vi "DQMH_API_OpenCreateEventDialog.vi"(8 "error in (no error)":errorcluster) -> (0 "error out":errorcluster, 3 "DqmhCreateEventDialogRef":refnum<vi>, 5 "ApplicationRef":refnum<vi>)   [LabVIEW 2016]
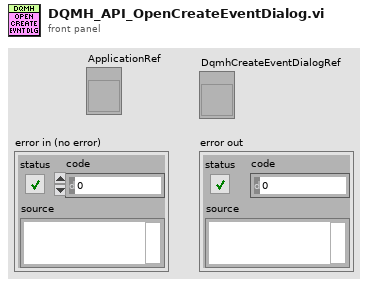
[diagram p1: front panel]
types:
  T1 = enum32{"Bad", "Idle", "Run top level", "Running"}
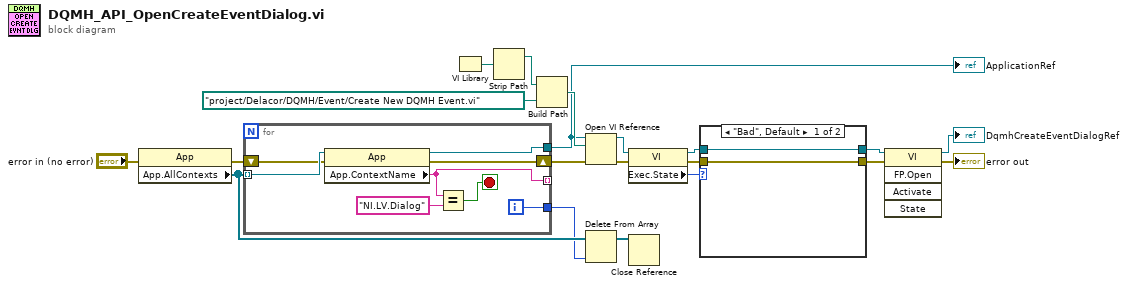
[diagram p0: block diagram]
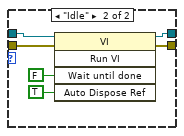
[diagram p2: hidden frame]
diagram:
  n1 = property class="App"(error in="error in (no error)") -> (error out=w18:errorcluster, "App.AllContexts"=w13:refnum<vi>[])  [unwired: 1 in, 1 out]
  n2 = for {
    tunnel: w13 -> [w28] mode=indexing
    tunnel: [w26] -> _ mode=indexing
    tunnel: [w24] -> w12
    tunnel: [w23] -> w1
    shift-right: [w22] -> w17
    shift-left: w18 -> [w21]
    i -> [w24]
    stop <- w25 stop-if-true
    n3 = property class="App"(reference=w28, error in=w21) -> (reference out=w23:refnum<vi>, error out=w22:errorcluster, "App.ContextName"=w26:string)
    n4 = Equal?(x=w26, y="NI.LV.Dialog" ("App.ContextName")) -> (x = y?=w25:bool)
  }
  "ApplicationRef" <- w1
  n5 = VI Library() -> (path=w10:path)
  n6 = Strip Path(path=w10) -> (stripped path=w9:path)  [unwired: 1 out]
  n7 = Build Path(base path=w9, name or relative path=path "project/Delacor/DQMH/Event/Create New DQMH Event.vi") -> (appended path=w7:path)
  n8 = Open VI Reference(application reference (local)=w1, vi path=w7, error in (no error)=w17) -> (vi reference=w6:refnum<vi>, error out=w5:errorcluster)  [unwired: 3 in]
  n9 = Delete From Array(array=w13, index=w12) -> (array with subset deleted=w11:refnum<vi>[])  [unwired: 1 in, 1 out]
  n10 = property class="VI"(reference=w6, error in=w5) -> (reference out=w3:refnum<vi>, error out=w16:errorcluster, "Exec.State"=w4:T1)
  n11 = Close Reference(reference=w11) -> ()  [unwired: 1 in, 1 out]
  n12 = case shown="\"Bad\", Default" w4 {
    tunnel: w3 -> [w30 w36]
    tunnel: [w30 w33] -> w2
    tunnel: [w29 w32] -> w15
    tunnel: w16 -> [w29 w31]
    frame "Bad", Default {
    }
    frame "Idle" {
      n13 = invoke class="VI" method="Run VI"(reference=w36, error in=w31, "Wait until done"=FALSE ("Wait Until Done"), "Auto Dispose Ref"=TRUE ("Wait Until Done")) -> (reference out=w33:refnum<vi>, error out=w32:errorcluster)  [unwired: 1 in, 3 out]
    }
  }
  n14 = invoke class="VI" method="FP.Open"(reference=w2, error in=w15) -> (reference out=→"DqmhCreateEventDialogRef":refnum<vi>, error out=→"error out":errorcluster)  [unwired: 3 in, 3 out]
